vi "Enable.vi"(11 "ChannelSetArray2":T1[](array[typedef]) {"Enable" items=["不使能", "使能"]; "Wave" items=["0指令", "正弦波", "方波", "三角波", "常值", "波形数据", "白噪声", "正弦扫频", "梯度加载", "VMIC"]; "ChannelType" items=["标准波形跟踪"=1, "扫频测试"=2, "消除多余力"=3, "梯度加载"=4, "载荷谱跟踪"=5, "模拟输入跟踪"=9]; "ChannelStatus" items=["通道关", "位置通道", "加载通道"]}) -> (3 "Enable":bool[](array[boolean]))   [LabVIEW 2014]
uses:
  ChannelCommand.ctl
  Control 1.ctl
  WaveType.ctl
  MoterEnable.ctl
panel:
  in  "Boolean 2":bool
  in  "Boolean":bool=TRUE
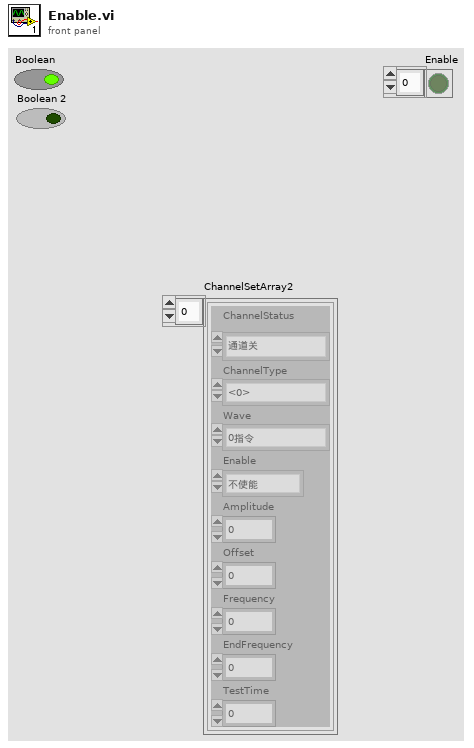
[diagram p1: front panel]
types:
  T1 = typedef "ChannelCommand.ctl" = cluster{"ChannelStatus":T2, "ChannelType":i32, "Wave":T3, "Enable":T4, "Amplitude":dbl, "Offset":dbl, "Frequency":dbl, "EndFrequency":dbl, "TestTime":dbl}
  T2 = typedef "Control 1.ctl" = i32
  T3 = typedef "WaveType.ctl" = i32
  T4 = typedef "MoterEnable.ctl" = u16
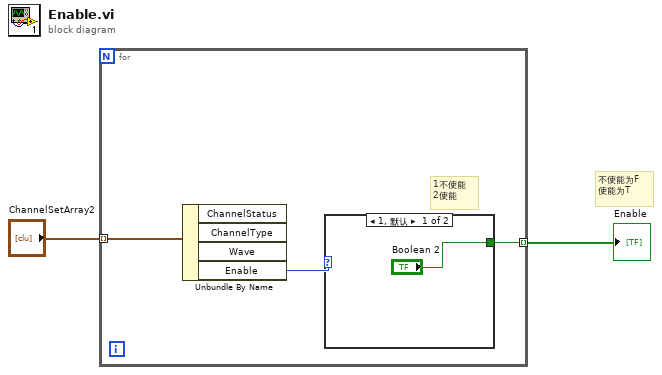
[diagram p0: block diagram]
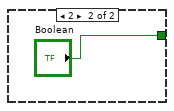
[diagram p2: hidden frame]
diagram:
  # "不使能为F\n使能为T"
  n1 = for {
    tunnel: "ChannelSetArray2" -> [w5] mode=indexing
    tunnel: [w3] -> w1 mode=indexing
    # "1不使能\n2使能"
    n2 = Unbundle By Name(w5) -> ("Enable"=w4:T4)  [unwired: 3 out]
    n3 = case shown="1, 默认" w4 {
      tunnel: ["Boolean 2" "Boolean"] -> w3
      frame 1, Default {
      }
      frame 2 {
      }
    }
  }
  "Enable" <- w1
